vi "DevB.Create Message Session.vi"(8 "error in":errorcluster, 10 "stop event":refnum<user-event>) -> (0 "error out":errorcluster, 2 "DevB Message queue":refnum<queue>, 3 "DevB Session out":T1)   [LabVIEW 2018]
uses:
  typedefs/DevB.Message.ctl
  typedefs/DevB.Message type.ctl
  typedefs/DevB.Message Session.ctl
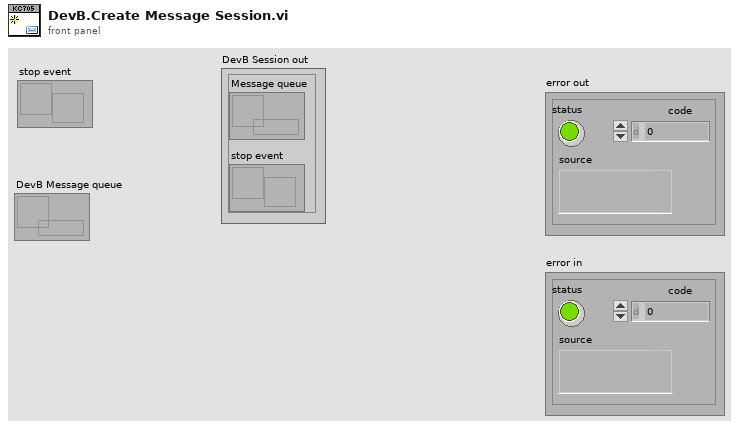
[diagram p1: front panel]
types:
  T1 = typedef "DevB.Message Session.ctl" = cluster{"Message queue":refnum<queue>, "stop event":refnum<user-event>}
  T2 = typedef "DevB.Message.ctl" = cluster{"type":T3, "data":variant}
  T3 = typedef "DevB.Message type.ctl" = enum16{"Idle", "Set Duration", "Set Frequency", "Set Phase", "Set Delay", "on/off", "check status"}
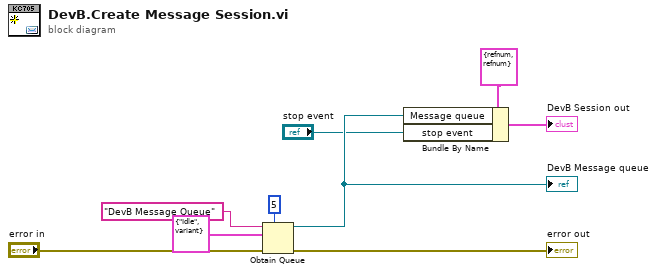
[diagram p0: block diagram]
diagram:
  n1 = Obtain Queue(max queue size (-1, unlimited)=5, name (unnamed)="DevB Message Queue", element data type=T2 {"type"=enum."Idle", "data"=variant} ("DevB.Message"), error in (no error)="error in") -> (queue out=w4:refnum<queue>, error out=→"error out":errorcluster)  [unwired: 1 in, 1 out]
  "DevB Message queue" <- w4
  n2 = Bundle By Name(cluster=T1 {"Message queue"=refnum, "stop event"=refnum} ("DevBoard Message session"), "Message queue"=w4, "stop event"="stop event") -> (→"DevB Session out":T1)
